vi "Measure.vi"(8 "error in (no error)":errorcluster, 11 "Scale in":refnum<class "Scale.lvclass">) -> (0 "error out":errorcluster, 2 "Mass":dbl[unit], 3 "Scale out":refnum<class "Scale.lvclass">)   [LabVIEW 2021, in "Scale.lvclass"]
uses:
  Scale.lvclass
  <vilib>/ptbypt/NI_PtbyPt.lvlib
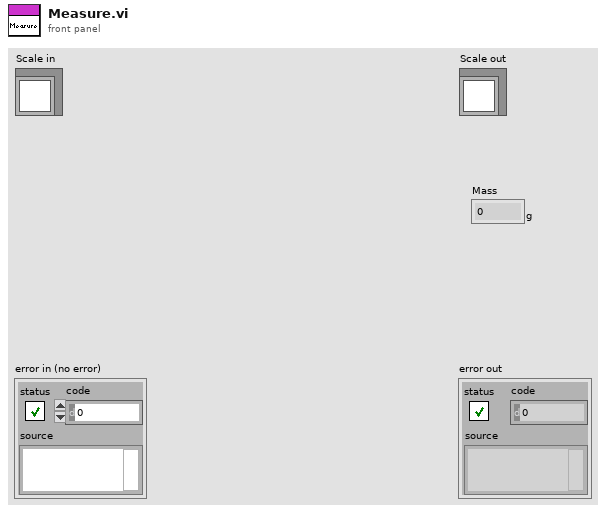
[diagram p1: front panel]
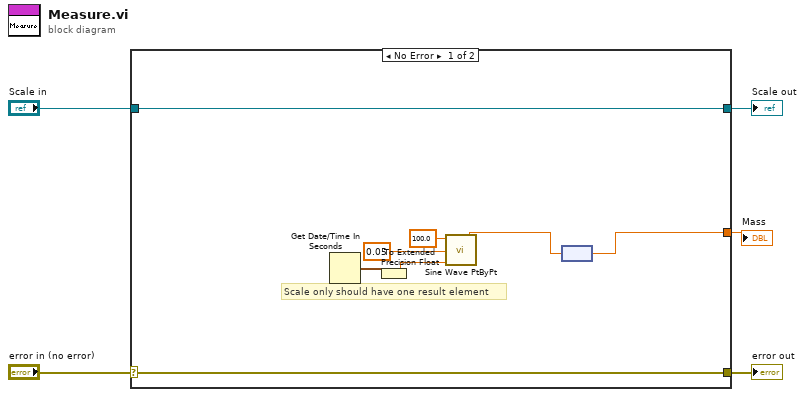
[diagram p0: block diagram]
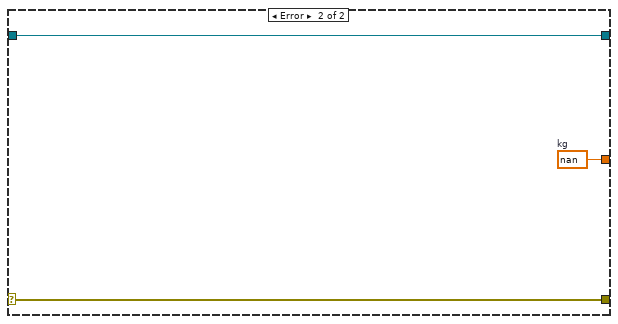
[diagram p2: hidden frame]
diagram:
  n1 = case shown="No Error" "error in (no error)" {
    selector: "error in (no error)" -> [w6 w16]
    tunnel: [w6 w16] -> w4
    tunnel: [w7 w15] -> w2
    tunnel: "Scale in" -> [w7 w15]
    tunnel: [w8 w14] -> w1
    frame No Error {
      # "Scale only should have one result element"
      n2 = Get Date/Time In Seconds() -> (seconds since 1Jan1904=w12:timestamp)
      n3 = To Extended Precision Float(1:w12) -> (0:w11:ext)
      n4 = call <vilib>:"Sine Wave PtByPt.vi"("time"=w11, "frequency"=0.05, "amplitude"=100.0) -> ("sine wave"=w9:dbl)  [unwired: 1 in]
      n5 = node(w9) -> (w8:dbl[unit])
    }
    frame Error {
      w14 = dbl[unit] nan  # kg
    }
  }
  "error out" <- w4
  "Scale out" <- w2
  "Mass" <- w1
